vi "crear_leer_ficherosXML.vi"() -> ()   [LabVIEW 2019]
panel:
  out "ARRAY CLUSTERS":T1(array[cluster])
  out "Cluster":T2
  out "nº celdas":u16
  out "Paso Y":dbl
  out "Paso X":dbl
  in  "nº celdas":u16
  in  "Paso Y":dbl
  in  "Paso X":dbl
  out "error out":errorcluster
  in  "error in (no error)":errorcluster
  in  "nombre bandeja":string
  in  "ancho":u32
  in  "largo":u32
  in  "alto":u32
  in  "Crear Bandeja?":bool
  out "ANCHO":u32
  out "LARGO":u32
  out "ALTO":u32
  out "filenames":string[](array[string])
  in  "SELECTOR BANDEJA":string(combo)
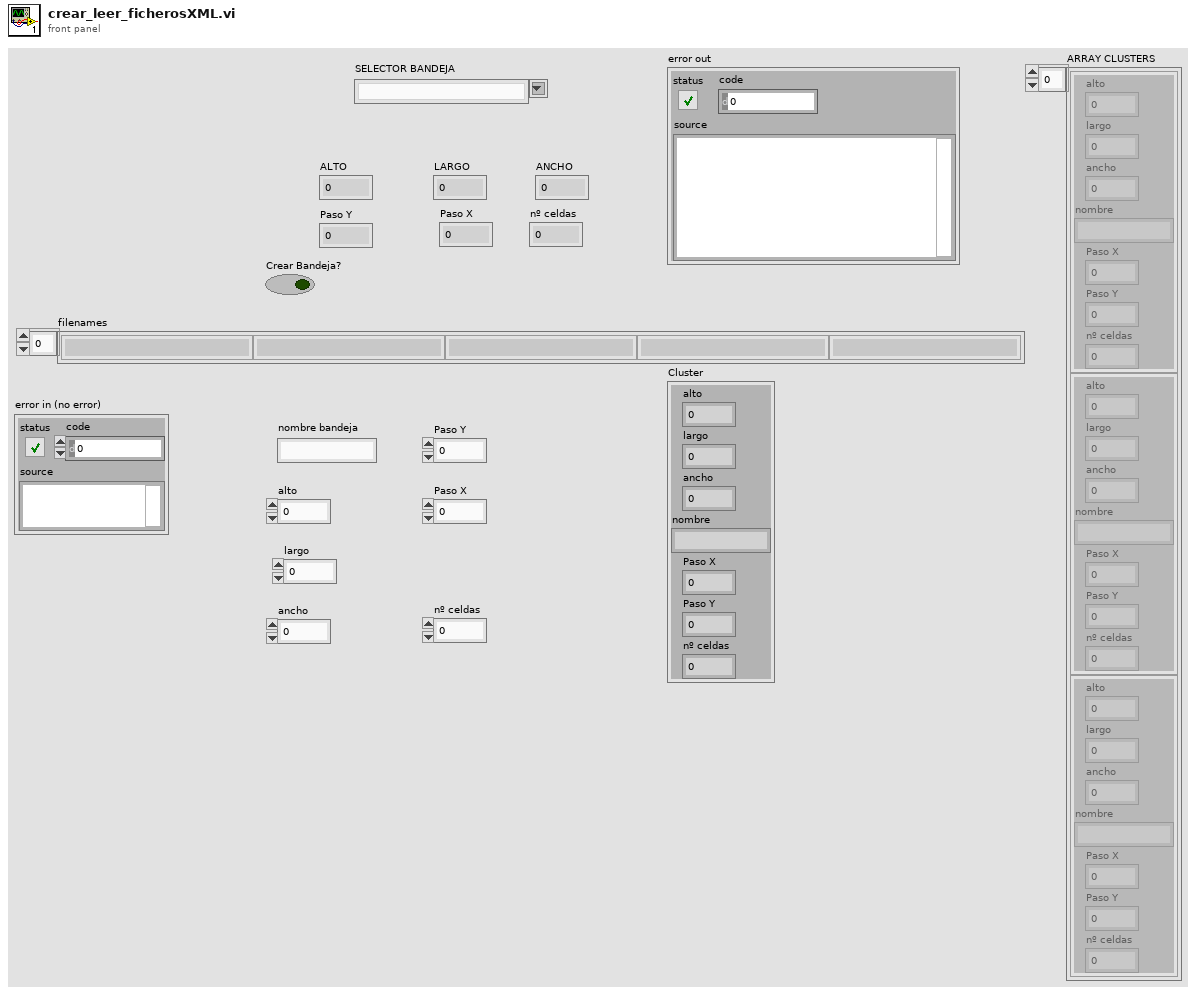
[diagram p1: front panel]
types:
  T1 = cluster{"alto":u32, "largo":u32, "ancho":u32, "nombre":string, "Paso X":dbl, "Paso Y":dbl, "nº celdas":u16}[]
  T2 = cluster{"alto":u32, "largo":u32, "ancho":u32, "nombre":string, "Paso X":dbl, "Paso Y":dbl, "nº celdas":u16}
  T3 = enum16{"Start", "Crear Bandeja Nueva?", "Datos validos?", "Crear bandeja", "Cargar Bandejas Actuales", "Leer Bandeja Escogida", "Error?", "Salir"}
  T4 = cluster{"Nº de columnas ":u16, "Nº de filas ":u16, "largo":u32, "ancho":u32, "nombre":string, "Paso X":dbl, "Paso Y":dbl, "DISTANCIA SUELO A CHIP  ":dbl, "Nº de celdas totales":u16, "Distancia chips bandejas contiguas":dbl}[]
  T5 = cluster{"Nº de columnas ":u16, "Nº de filas ":u16, "largo":u32, "ancho":u32, "nombre":string, "Paso X":dbl, "Paso Y":dbl, "DISTANCIA SUELO A CHIP  ":dbl, "Nº de celdas totales":u16, "Distancia chips bandejas contiguas":dbl}
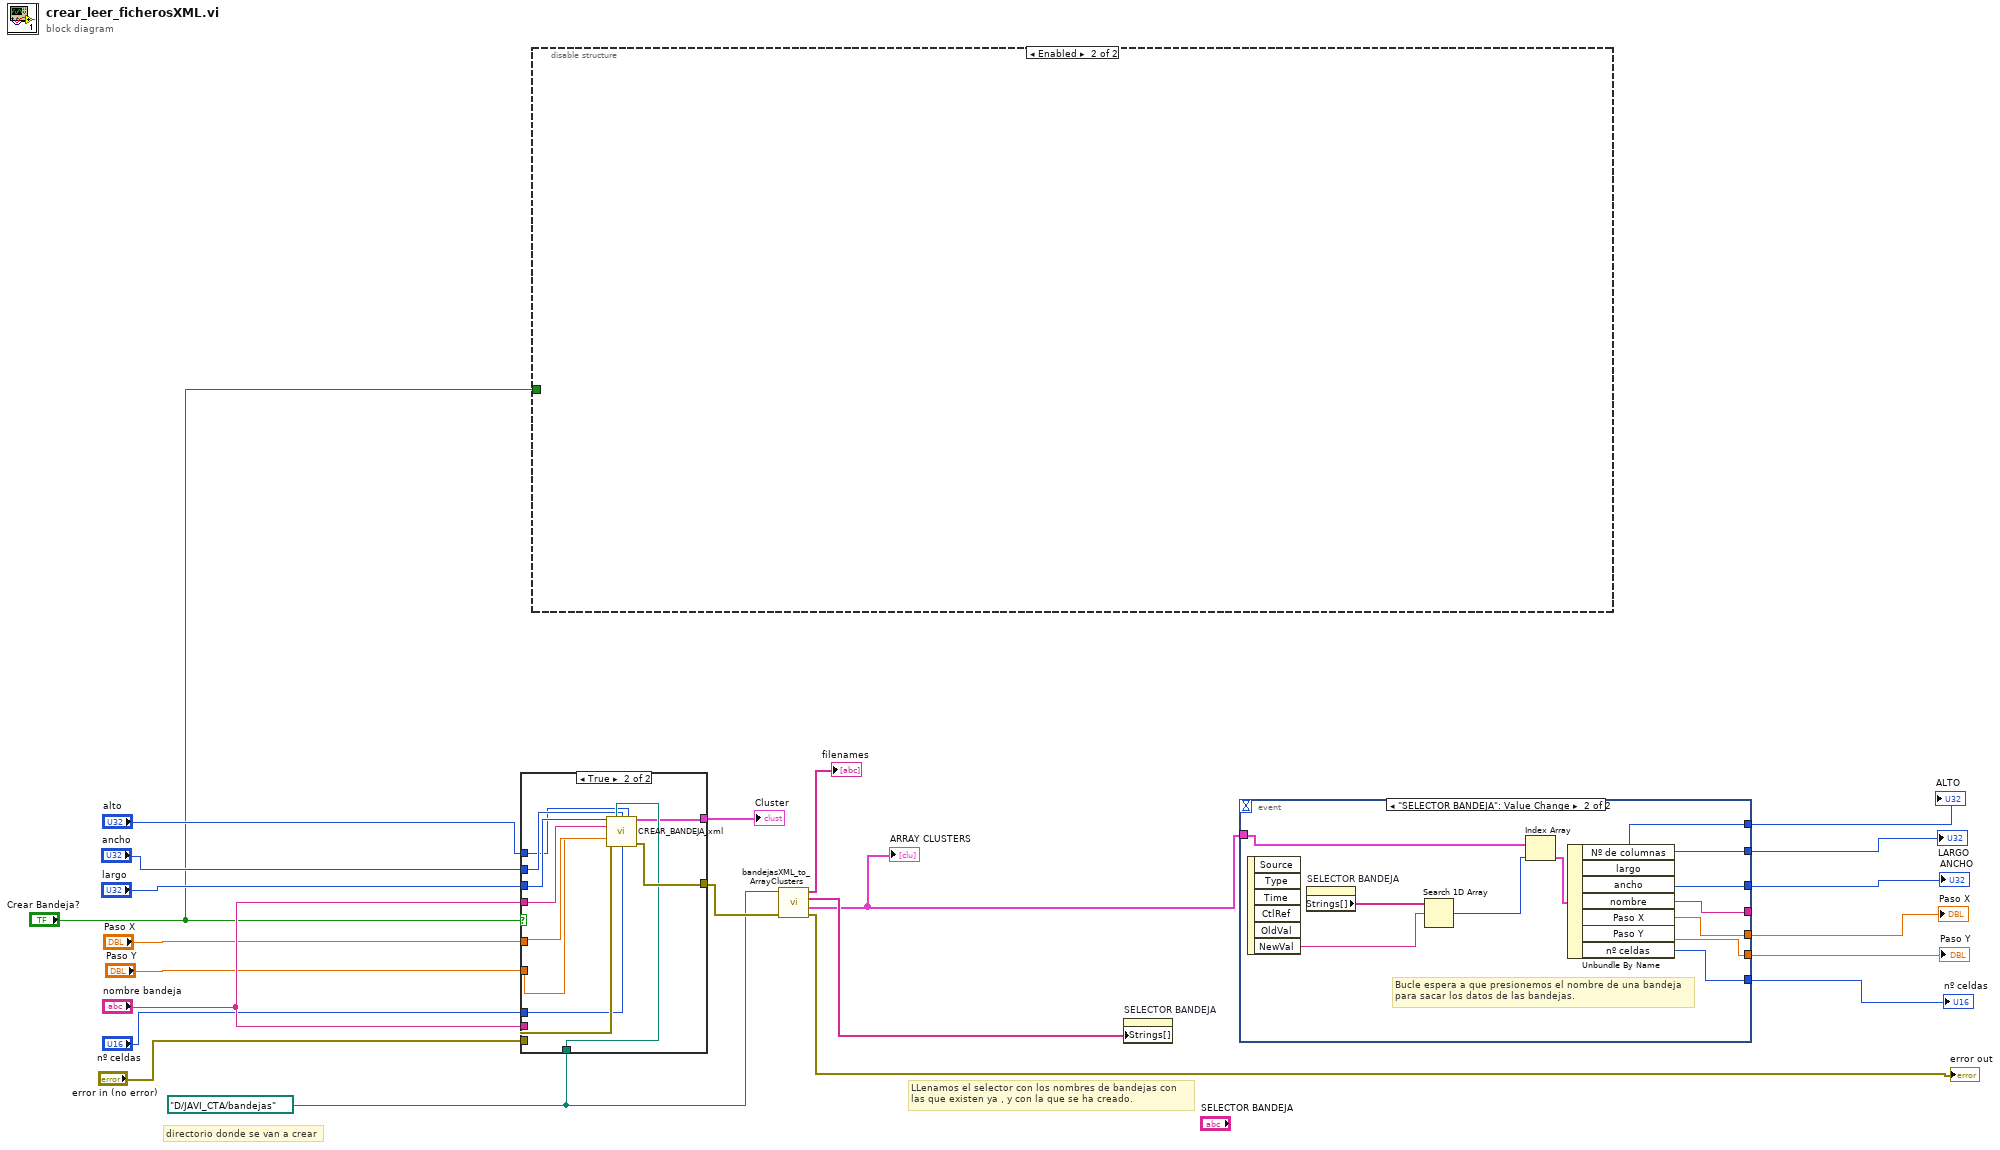
[diagram p0: block diagram]
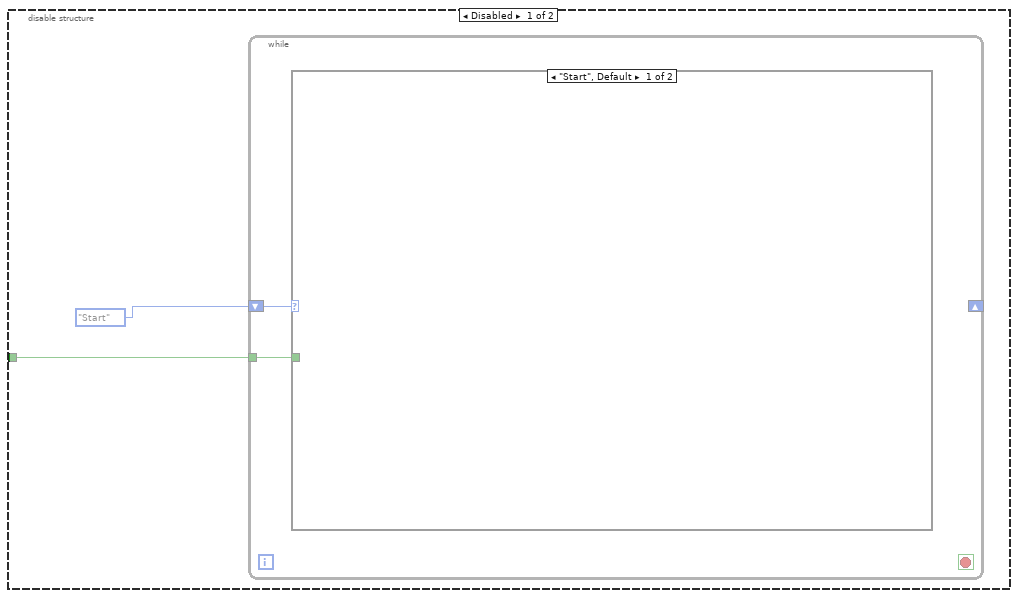
[diagram p2: hidden frame]
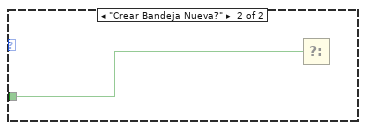
[diagram p3: hidden frame]
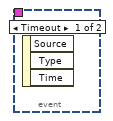
[diagram p5: hidden frame]
diagram:
  w21 = path "D:/JAVI_CTA/bandejas" ("path")
  # "LLenamos el selector con los nombres de bandejas con \nlas que existen ya , y con la que se ha creado."
  # "directorio donde se van a crear"
  n1 = case shown="True" "Crear Bandeja?" {
    tunnel: [w23 w34] -> w22
    tunnel: w21 -> [_ w33]
    tunnel: "alto" -> [_ w29]
    tunnel: "ancho" -> [_ w30]
    tunnel: "largo" -> [_ w31]
    tunnel: "nombre bandeja" -> [_ _]
    tunnel: "nombre bandeja" -> [_ w32]
    tunnel: "error in (no error)" -> [w23 w28]
    tunnel: "Paso X" -> [_ w27]
    tunnel: "Paso Y" -> [_ w25]
    tunnel: "nº celdas" -> [_ w26]
    tunnel: [_ w24] -> w3
    frame False {
    }
    frame True {
      n2 = call "CREAR_BANDEJA_xml.vi"("largo"=w31, "path"=w33, "ancho"=w30, "alto"=w29, "nombre bandeja"=w32, "Paso X"=w27, "error in (no error)"=w28, "Paso Y"=w25, "nº celdas"=w26) -> ("Cluster"=w24:T2, "error out"=w34:errorcluster)  [unwired: 5 in]
    }
  }
  "Cluster" <- w3
  n3 = disable-structure shown="Enabled" {
    disable-tunnel: "Crear Bandeja?" -> [w35 _]
    frame Disabled {
      n4 = while {
        shift-right: _ -> [_]
        shift-left: T3."Start" -> [w38]
        tunnel: w35 -> [w37]
        stop <- _ stop-if-true
        n5 = case shown="\"Start\", Default" w38 {
          tunnel: w37 -> [_ w39]
          frame "Start", Default {
          }
          frame "Crear Bandeja Nueva?" {
            n6 = Select(s=w39) -> ()  [unwired: 2 in, 1 out]
          }
        }
      }
    }
    frame Enabled {
    }
  }
  n7 = call "bandejasXML_to_ArrayClusters.vi"("error in (no error)"=w22, "path"=w21) -> ("error out"=→"error out":errorcluster, "Array Clusters Bandejas"=w1:T4, "filenames"=→"filenames":string[], "Nombres bandejas"=w20:string[])  [unwired: 6 in]
  "ARRAY CLUSTERS" <- w1
  n8 = property on="SELECTOR BANDEJA" class="CmbBox"("Strings[]"=w20) -> ()  [unwired: 2 in, 2 out]
  n9 = event shown="[1] \"SELECTOR BANDEJA\": Value Change" {
    selector: _ -> [_ _]
    dyn-events: _ -> [_ _]
    timeout: _ -> [_ _]
    tunnel: [_ w47] -> w9
    tunnel: [_ w46] -> w8
    tunnel: [_ w45] -> w7
    tunnel: [_ w44] -> _
    tunnel: [_ w43] -> w6
    tunnel: [_ w42] -> w5
    tunnel: [_ w41] -> w4
    tunnel: w1 -> [_ w40]
    event Timeout {
      n10 = event-data() -> ()  [unwired: 1 in, 3 out]
    }
    event "SELECTOR BANDEJA": Value Change {
      # "Bucle espera a que presionemos el nombre de una bandeja\npara sacar los datos de las bandejas."
      n11 = event-data() -> ("NewVal"=w50:string)  [unwired: 1 in, 5 out]
      n12 = property on="SELECTOR BANDEJA" class="CmbBox"() -> ("Strings[]"=w51:string[])  [unwired: 2 in, 2 out]
      n13 = Search 1D Array(1D array=w51, element=w50) -> (index of element=w49:i32)  [unwired: 1 in]
      n14 = Index Array(array=w40, index=w49) -> (element=w48:T5)
      n15 = Unbundle By Name(w48) -> ("Nº de columnas"=w47:u16, "largo"=w46:u32, "ancho"=w45:u32, "nombre"=w44:string, "Paso X"=w43:dbl, "Paso Y"=w42:dbl, "nº celdas"=w41:u16)
    }
  }
  "ALTO" <- w9
  "LARGO" <- w8
  "ANCHO" <- w7
  "Paso X" <- w6
  "Paso Y" <- w5
  "nº celdas" <- w4
